vi "Move In Previous Page.vi"(8 "error in (no error)":errorcluster, 11 "Test Channel View in":refnum<class "HVAC System View.lvclass">) -> (0 "error out":errorcluster, 3 "Test Channel View out":refnum<class "HVAC System View.lvclass">)   [LabVIEW 2013, in "HVAC System View.lvlib" / "HVAC System View.lvclass"]
uses:
  HVAC System View.lvclass
  HVAC System View.lvclass/HVAC System View.ctl
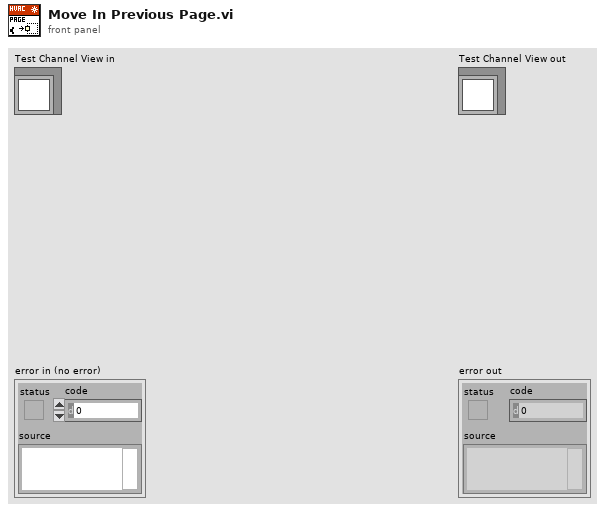
[diagram p1: front panel]
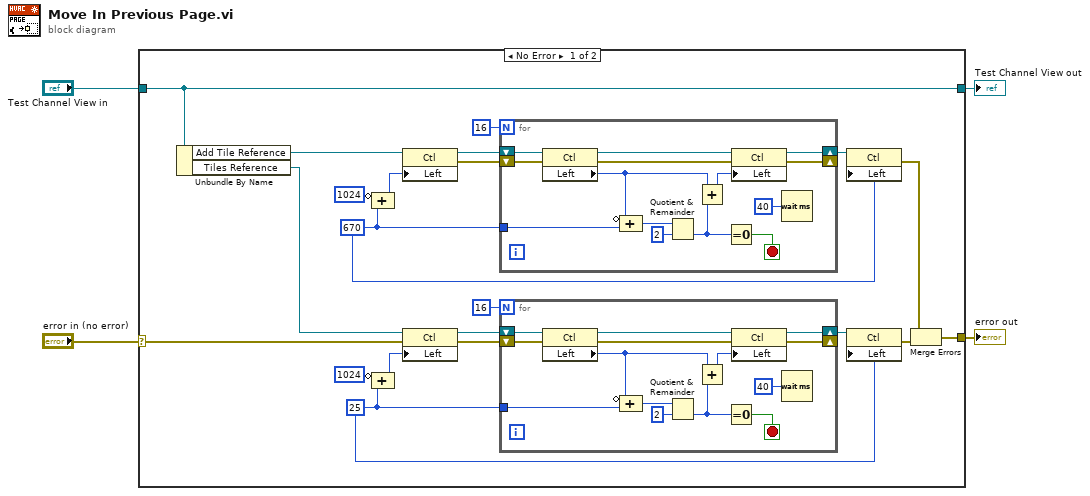
[diagram p0: block diagram]
diagram:
  n1 = case shown="No Error" "error in (no error)" {
    selector: "error in (no error)" -> [w16 w55]
    tunnel: "Test Channel View in" -> [w10 w54]
    tunnel: [w12 w55] -> w1
    tunnel: [w10 w54] -> w3
    frame No Error {
      w5 = 25 ("Splitter Position")
      w7 = 670 ("Splitter Position")
      n2 = Unbundle By Name(w10) -> ("Add Tile Reference"=w24:refnum<vi>, "Tiles Reference"=w17:refnum<vi>)
      n3 = Compound Arithmetic op=unknown(invert 1024 ("Position:Left"), w7) -> (w23:i32)
      n4 = Compound Arithmetic op=unknown(invert 1024 ("Position:Left"), w5) -> (w18:i32)
      n5 = property class="Ctl"(reference=w24, "Left"=w23) -> (reference out=w22:refnum<vi>, error out=w14:errorcluster)  [unwired: 1 in]
      n6 = property class="Ctl"(reference=w17, error in=w16, "Left"=w18) -> (reference out=w19:refnum<vi>, error out=w15:errorcluster)
      n7 = for {
        N: 16 -> [_]
        shift-right: [w51] -> w21
        shift-left: w22 -> [w53]
        shift-right: [w44] -> _
        shift-left: w14 -> [w52]
        tunnel: w7 -> [w40]
        stop <- w43 stop-if-true
        n8 = property class="Ctl"(reference=w53, error in=w52) -> (reference out=w49:refnum<vi>, error out=w50:errorcluster, "Left"=w41:i32)
        n9 = Compound Arithmetic op=ADD(invert w41, w40) -> (w47:i32)
        n10 = Quotient & Remainder(x=w47, y=2) -> (floor(x/y)=w45:i32)  [unwired: 1 out]
        n11 = Add(x=w41, y=w45) -> (x+y=w48:i32)
        n12 = Equal To 0?(x=w45) -> (x = 0?=w43:bool)
        n13 = property class="Ctl"(reference=w49, error in=w50, "Left"=w48) -> (reference out=w51:refnum<vi>, error out=w44:errorcluster)
        n14 = Wait (ms)(milliseconds to wait=u32 40) -> ()  [unwired: 1 out]
      }
      n15 = for {
        N: 16 -> [_]
        shift-right: [w37] -> w20
        shift-left: w19 -> [w39]
        shift-right: [w30] -> _
        shift-left: w15 -> [w38]
        tunnel: w5 -> [w26]
        stop <- w29 stop-if-true
        n16 = property class="Ctl"(reference=w39, error in=w38) -> (reference out=w35:refnum<vi>, error out=w36:errorcluster, "Left"=w27:i32)
        n17 = Compound Arithmetic op=ADD(invert w27, w26) -> (w33:i32)
        n18 = Quotient & Remainder(x=w33, y=2) -> (floor(x/y)=w31:i32)  [unwired: 1 out]
        n19 = Add(x=w27, y=w31) -> (x+y=w34:i32)
        n20 = Equal To 0?(x=w31) -> (x = 0?=w29:bool)
        n21 = property class="Ctl"(reference=w35, error in=w36, "Left"=w34) -> (reference out=w37:refnum<vi>, error out=w30:errorcluster)
        n22 = Wait (ms)(milliseconds to wait=u32 40) -> ()  [unwired: 1 out]
      }
      n23 = property class="Ctl"(reference=w21, "Left"=w7) -> (error out=w11:errorcluster)  [unwired: 1 in, 1 out]
      n24 = property class="Ctl"(reference=w20, "Left"=w5) -> (error out=w13:errorcluster)  [unwired: 1 in, 1 out]
      n25 = Merge Errors(w11, w13) -> (w12:errorcluster)
    }
    frame Error {
    }
  }
  "error out" <- w1
  "Test Channel View out" <- w3
